vi "SIFS_Receive.vi"(4 "error in":errorcluster, 5 "Command to SIFS":string, 6 "wait after tx":u32, 7 "VISA resource name":refnum<visa-resource-name>) -> (0 "error out":errorcluster, 1 "cmd sent":bool, 2 "Response from SIFS":string, 3 "VISA resource name out":refnum<visa-resource-name>)   [LabVIEW 2012]
uses:
  GLOBAL.vi
panel:
  out "error out 2":errorcluster
  out "error IO":errorcluster
  out "Numeric":i32
  out "read buffer":string
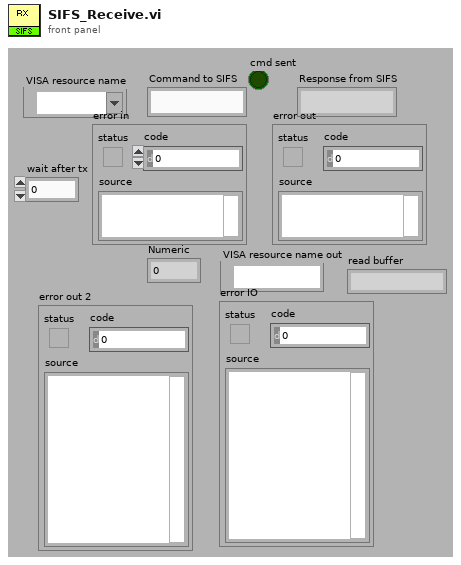
[diagram p1: front panel]
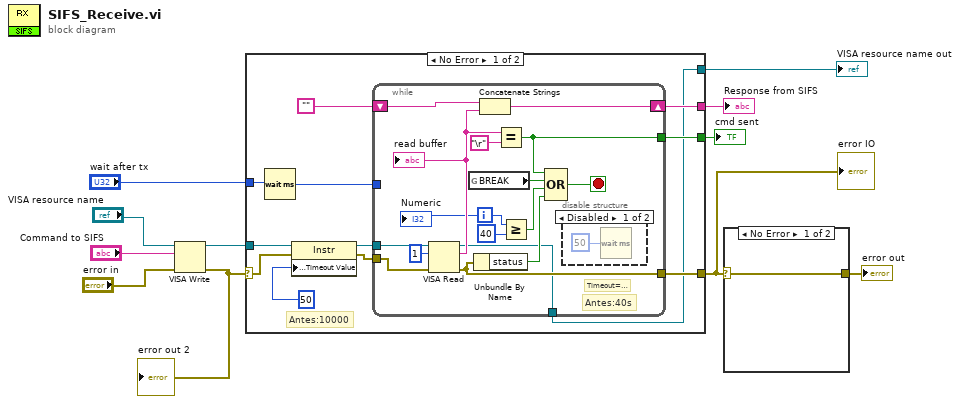
[diagram p0: block diagram]
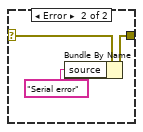
[diagram p2: hidden frame]
diagram:
  n1 = VISA Write(VISA resource name="VISA resource name", write buffer="Command to SIFS", error in (no error)="error in") -> (VISA resource name out=w9:refnum<visa-resource-name>, error out=w8:errorcluster)  [unwired: 1 out]
  "error out 2" <- w8
  n2 = case shown="No Error" w8 {
    selector: w8 -> [w13 w42]
    tunnel: [w19 w42] -> w6
    tunnel: [w23 _] -> w11
    tunnel: w9 -> [w16 w41]
    tunnel: "wait after tx" -> [w20 _]
    tunnel: [w18 _] -> w4
    tunnel: [w12 w41] -> w1
    frame No Error {
      # "Antes:10000"
      n3 = Wait (ms)(milliseconds to wait=w20) -> (millisecond timer value=w21:u32)
      n4 = property class="Instr"(reference=w16, error in=w13, "General Settings:Timeout Value"=u32 50) -> (reference out=w15:refnum<visa-resource-name>, error out=w14:errorcluster)
      n5 = while {
        shift-right: [w38] -> w23
        shift-left: "" -> [w39]
        tunnel: [w28] -> w19
        tunnel: w21 -> [_]
        tunnel: [w27] -> w18
        tunnel: w15 -> [w26]
        tunnel: w14 -> [w25]
        tunnel: [w24] -> w12
        i -> [w32]
        stop <- w33 stop-if-true
        # "Antes:40s"
        # "Timeout=2s"
        n6 = VISA Read(VISA resource name=w26, byte count=u32 1, error in (no error)=w25) -> (VISA resource name out=w24:refnum<visa-resource-name>, read buffer=w35:string, error out=w28:errorcluster)  [unwired: 1 out]
        "read buffer" <- w35
        n7 = global read "GLOBAL.vi" "BREAK"() -> (w34:bool)
        n8 = Unbundle By Name(w28) -> ("status"=w29:bool)
        n9 = Concatenate Strings(w39, w35) -> (w38:string)
        n10 = Equal?(x=w35, y="\r") -> (x = y?=w27:bool)
        n11 = Greater Or Equal?(x=w32, y=40) -> (x >= y?=w30:bool)
        n12 = Compound Arithmetic op=OR(w27, w34, w30, w29) -> (w33:bool)
        n13 = disable-structure shown="Disabled" {
          frame Disabled {
            n14 = Wait (ms)(milliseconds to wait=u32 50 ("millisecond multiple")) -> ()  [unwired: 1 out]
          }
          frame Enabled {
          }
        }
        "Numeric" <- w32
      }
    }
    frame Error {
    }
  }
  "Response from SIFS" <- w11
  "VISA resource name out" <- w1
  "cmd sent" <- w4
  "error IO" <- w6
  n15 = case shown="No Error" w6 {
    selector: w6 -> [w43 w45]
    tunnel: [w43 w44] -> w5
    frame No Error {
    }
    frame Error {
      n16 = Bundle By Name(cluster=w45, "source"="Serial error") -> (w44:errorcluster)
    }
  }
  "error out" <- w5
